vi "Convert Error Cluster to Table.vi"(11 "Error Codes":cluster{i32, string}[](array[cluster])) -> (2 "Code":i32[](array[numeric]), 3 "String":string[](array[string]))   [LabVIEW 2019, in "Diagnostics Addon System Explorer.lvlib"] (continued)
additional write network transactions can occur."}, {-40618, "LabVIEW: (Hex 0xFFFF6156) The reference is invalid."}, {-40616, "LabVIEW: (Hex 0xFFFF6158) The deterministic communication engine is unable to locate a device with a specified MAC address."}, {-40615, "LabVIEW: (Hex 0xFFFF6159) LabVIEW cannot instantiate the requested device in a specified mode because there is already a device initialized in deterministic mode."}, {-40613, "LabVIEW: (Hex 0xFFFF615B) The specified subchannel is out of range.  Refer to the LabVIEW Help for more information about supported ranges for channel subchannels."}, {-40612, "LabVIEW: (Hex 0xFFFF615C) You have attempted one of the following illegal operations: allocation of a write terminal on a channel that another node owns; allocation of a shared memory variable on a non-shared memory channel; creation of a read or write terminal on a shared memory channel."}, {-40611, "LabVIEW: (Hex 0xFFFF615D) An item with the specified index has already been configured."}, {-40609, "LabVIEW: (Hex 0xFFFF615F) The item offset is outside of the range you specified during channel initialization time."}, {-40608, "LabVIEW: (Hex 0xFFFF6160) One of the following occurred: 1) Message being written to the deterministic-communication engine exceeds the maximum size configured when the channel or terminal was created. 2) Buffer allocated for reading is smaller than the message size."}, {-40606, "LabVIEW: (Hex 0xFFFF6162) A timing source with the same name already exists for the deterministic-communication engine."}, {-40603, "LabVIEW: (Hex 0xFFFF6165) Files for the deterministic-communication engine are not installed properly."}, {-40602, "LabVIEW: (Hex 0xFFFF6166) Deterministic-communication engine ran out of allocated resources."}, {-40601, "LabVIEW: (Hex 0xFFFF6167) The deterministic-communication engine failed to initialize hardware."}, {-40600, "LabVIEW: (Hex 0xFFFF6168) The deterministic communication engine failed to allocate enough memory while performing the requested operation."}, {-36517, "LabVIEW: (Hex 0xFFFF715B) MathScript cannot execute a function which is overwritten by a variable in other code branches."}, {-36516, "LabVIEW: (Hex 0xFFFF715C) The variable is undefined. Assign a value to the variable before read access occurs."}, {-36515, "LabVIEW: (Hex 0xFFFF715D) Accessing a structure field is only supported for scalar structures but not for structure arrays."}, {-36514, "LabVIEW: (Hex 0xFFFF715E) Argument must be a positive integer scalar."}, {-36513, "LabVIEW: (Hex 0xFFFF715F) User-defined error message:"}, {-36512, "LabVIEW: (Hex 0xFFFF7160) Output data lost due to converting a non-vector character array to a string."}, {-36511, "LabVIEW: (Hex 0xFFFF7161) The result is not applicable because it returned a complex integer data type, which is not supported."}, {-36510, "LabVIEW: (Hex 0xFFFF7162) The switch selector must be a scalar."}, {-36509, "LabVIEW: (Hex 0xFFFF7163) The complete evaluation of a short-circuit expression detected a semantic error."}, {-36508, "LabVIEW: (Hex 0xFFFF7164) You must use an argument with a scalar value that can be converted into a logical value."}, {-36507, "LabVIEW: (Hex 0xFFFF7165) Converting a multi-element array into a scalar value resulted in lost output data."}, {-36506, "LabVIEW: (Hex 0xFFFF7166) Converting a complex number with non-zero imaginary values into a real number resulted in lost output data."}, {-36505, "LabVIEW: (Hex 0xFFFF7167) The argument types are not supported."}, {-36504, "LabVIEW: (Hex 0xFFFF7168) You cannot output an empty array as a scalar value."}, {-36503, "LabVIEW: (Hex 0xFFFF7169) The arguments must have matching dimensions to replace the indexing of an array."}, {-36502, "LabVIEW: (Hex 0xFFFF716A) The index is out of bounds."}, {-36501, "LabVIEW: (Hex 0xFFFF716B) The arguments must be positive integers or logicals."}, {-36500, "LabVIEW: (Hex 0xFFFF716C) The arguments must have matching dimensions to build an array."}, {-20339, "LabVIEW: (Hex 0xFFFFB08D) There must be a signal wired to each input signal terminal."}, {-10856, "LabVIEW: (Hex 0xFFFFD598) An unexpected error occurred from the operating system while performing the given operation."}, {-10846, "LabVIEW: (Hex 0xFFFFD5A2) Your application was unable to retrieve data from the background acquisition buffer fast enough so the unretrieved data was overwritten with new data.  To prevent this error, you might increase the size of the background acquisition buffer, increase the amount of data you read from it per call to the read function/VI, slow down your acquisition rate, or reduce the number of tasks your computer is performing."}, {-10804, "LabVIEW: (Hex 0xFFFFD5CC) The transfer stopped prior to reaching the end of the transfer buffer."}, {-10444, "LabVIEW: (Hex 0xFFFFD734) No more system memory is available on the heap, or no more memory is available on the device, or insufficient disk space is available."}, {-10408, "LabVIEW: (Hex 0xFFFFD758) The specified channel is in use."}, {-10405, "LabVIEW: (Hex 0xFFFFD75B) No channel is available."}, {-10403, "LabVIEW: (Hex 0xFFFFD75D) The specified device does not support the requested action (the driver recognizes the device, but the action is inappropriate for the device)."}, {-10402, "LabVIEW: (Hex 0xFFFFD75E) No device is located in the specified slot or at the specified address."}, {-10240, "LabVIEW: (Hex 0xFFFFD800) The driver interface could not locate or open the driver."}, {-10005, "LabVIEW: (Hex 0xFFFFD8EB) The device is invalid."}, {-10003, "LabVIEW: (Hex 0xFFFFD8ED) The value of a numeric parameter is invalid."}, {-4850, "LabVIEW: (Hex 0xFFFFED0E) Device driver not present or not supported."}, {-4824, "LabVIEW: (Hex 0xFFFFED28) Clipped Floating-point data to fit the range [-1.0, 1.0]."}, {-4820, "LabVIEW: (Hex 0xFFFFED2C) A buffer underflow has occurred."}, {-4803, "LabVIEW: (Hex 0xFFFFED3D) The sound driver or card does not support the specified operation."}, {-4702, "LabVIEW: (Hex 0xFFFFEDA2) One of the string parameters contains a null character. LabVIEW does not support null characters for regular expression matching."}, {-4701, "LabVIEW: (Hex 0xFFFFEDA3) The maximum recursion limit was reached while attempting the regular expression match"}, {-4644, "LabVIEW: (Hex 0xFFFFEDDC) An invalid UTF-8 string was used in a regular expression or input string."}, {-4643, "LabVIEW: (Hex 0xFFFFEDDD) Two named groups have the same name."}, {-4642, "LabVIEW: (Hex 0xFFFFEDDE) There is a syntax error after (?P."}, {-4641, "LabVIEW: (Hex 0xFFFFEDDF) An unrecognized character was encountered after (?P."}, {-4640, "LabVIEW: (Hex 0xFFFFEDE0) A recursive call could loop indefinitely."}, {-4639, "LabVIEW: (Hex 0xFFFFEDE1) Closing ) for (?C expected."}, {-4638, "LabVIEW: (Hex 0xFFFFEDE2) Number after (?C is > 255."}, {-4637, "LabVIEW: (Hex 0xFFFFEDE3) PCRE does not support \\L, \\l, \\N, \\P, \\p, \\U, \\u, or \\X escape sequences."}, {-4636, "LabVIEW: (Hex 0xFFFFEDE4) The \\C expression is not allowed in a lookbehind assertion."}, {-4635, "LabVIEW: (Hex 0xFFFFEDE5) Invalid condition (?(0)."}, {-4634, "LabVIEW: (Hex 0xFFFFEDE6) The character value in the \\x{...} sequence is too large."}, {-4632, "LabVIEW: (Hex 0xFFFFEDE8) UTF-8 is not supported."}, {-4631, "LabVIEW: (Hex 0xFFFFEDE9) POSIX collating elements are not supported."}, {-4630, "LabVIEW: (Hex 0xFFFFEDEA) Unknown POSIX class name."}, {-4629, "LabVIEW: (Hex 0xFFFFEDEB) A (?R or (?digits expression must be followed by )."}, {-4628, "LabVIEW: (Hex 0xFFFFEDEC) An assertion is expected after (?(."}, {-4627, "LabVIEW: (Hex 0xFFFFEDED) A conditional group contains more than two branches."}, {-4626, "LabVIEW: (Hex 0xFFFFEDEE) There is a malformed number after (?(."}, {-4625, "LabVIEW: (Hex 0xFFFFEDEF) A lookbehind assertion is not a fixed length."}, {-4624, "LabVIEW: (Hex 0xFFFFEDF0) The regular expression contains an unrecognized character after (?<."}, {-4623, "LabVIEW: (Hex 0xFFFFEDF1) Internal error: code overflow."}, {-4622, "LabVIEW: (Hex 0xFFFFEDF2) There is an unmatched parenthesis in a regular expression."}, {-4621, "LabVIEW: (Hex 0xFFFFEDF3) Failed to get the memory for regular expression matching."}, {-4620, "LabVIEW: (Hex 0xFFFFEDF4) The regular expression is too large."}, {-4619, "LabVIEW: (Hex 0xFFFFEDF5) Parentheses are nested too deeply."}, {-4618, "LabVIEW: (Hex 0xFFFFEDF6) A ) is missing after a comment."}, {-4617, "LabVIEW: (Hex 0xFFFFEDF7) Internal Error: Unknown option bit(s) set."}, {-4616, "LabVIEW: (Hex 0xFFFFEDF8) Internal Error: Erroffset passed as NULL."}, {-4615, "LabVIEW: (Hex 0xFFFFEDF9) There is a reference to non-existent subpattern."}, {-4614, "LabVIEW: (Hex 0xFFFFEDFA) A   ) is missing."}, {-4613, "LabVIEW: (Hex 0xFFFFEDFB) POSIX named classes are supported only within a class."}, {-4612, "LabVIEW: (Hex 0xFFFFEDFC) There is an unrecognized character after (?."}, {-4611, "LabVIEW: (Hex 0xFFFFEDFD) Internal error: unexpected repeat."}, {-4609, "LabVIEW: (Hex 0xFFFFEDFF) There is nothing to repeat."}, {-4608, "LabVIEW: (Hex 0xFFFFEE00) A range is out of order in a character class."}, {-4607, "LabVIEW: (Hex 0xFFFFEE01) A character class contains an invalid escape sequence."}, {-4606, "LabVIEW: (Hex 0xFFFFEE02) A character class is missing a ']' terminator."}, {-4605, "LabVIEW: (Hex 0xFFFFEE03) A number in the {} quantifier is too large."}, {-4604, "LabVIEW: (Hex 0xFFFFEE04) In the regular expression, the numbers within the quantifier {} are out of order."}, {-4603, "LabVIEW: (Hex 0xFFFFEE05) An unrecognized character follows a '\\'."}, {-4602, "LabVIEW: (Hex 0xFFFFEE06) A regular expression must not end with '\\c'. You must follow a '\\c' in a regular expression by another character to denote a control character."}, {-4601, "LabVIEW: (Hex 0xFFFFEE07) A regular expression must not end with '\\'."}, {-4600, "LabVIEW: (Hex 0xFFFFEE08) An unknown error occurred during the regular expression match."}, {-4550, "LabVIEW: (Hex 0xFFFFEE3A) This build specification uses VIs from a third party toolkit which is currently in evaluation mode."}, {-4502, "LabVIEW: (Hex 0xFFFFEE6A) A component of the given name is already loaded."}, {-4501, "LabVIEW: (Hex 0xFFFFEE6B) Cannot deploy without compiled code. Modify the build specification to include compiled code on the Additional Exclusions page before deploying."}, {-4407, "LabVIEW: (Hex 0xFFFFEEC9) LabVIEW cannot locate a palette item."}, {-4406, "LabVIEW: (Hex 0xFFFFEECA) A VI item in the <b>palette data</b> array is not supported in this version of LabVIEW."}, {-4404, "LabVIEW: (Hex 0xFFFFEECC) The value for <b>palette width</b> is invalid."}, {-4403, "LabVIEW: (Hex 0xFFFFEECD) A palette item is invalid."}, {-4402, "LabVIEW: (Hex 0xFFFFEECE) The palette view format is invalid."}, {-4401, "LabVIEW: (Hex 0xFFFFEECF) The specified file is not a valid palette file (.mnu)."}, {-4400, "LabVIEW: (Hex 0xFFFFEED0) The <b>palette type</b> is invalid."}, {-2985, "LabVIEW: (Hex 0xFFFFF457) The LabVIEW project is configured not to use source control. You must enable source control in order to perform source control operations."}, {-2984, "LabVIEW: (Hex 0xFFFFF458) The source control settings for the LabVIEW project require a different source control provider than what is configured for the LabVIEW environment. Select <b>Tools>>Source Control>>Configure Source Control</b> to change the source control provider for the LabVIEW environment."}, {-2983, "LabVIEW: (Hex 0xFFFFF459) LabVIEW could not access the source control provider. The LabVIEW source control configuration settings are not valid for this session or a timeout occurred. Select <b>Tools>>Source Control>>Configure Source Control</b> to reconfigure source control."}, {-2982, "LabVIEW: (Hex 0xFFFFF45A) The specified file is not a valid LabVIEW file type. Enter a path to an existing LabVIEW file, such as a VI or control."}, {-2981, "LabVIEW: (Hex 0xFFFFF45B) An error occurred while comparing the specified file. The local file is not the latest version in source control."}, {-2980, "LabVIEW: (Hex 0xFFFFF45C) The value of an input parameter is out of range."}, {-2979, "LabVIEW: (Hex 0xFFFFF45D) The source control configuration data is invalid, corrupted, or missing. Verify that the data is valid for the source control provider you selected during configuration."}, {-2978, "LabVIEW: (Hex 0xFFFFF45E) The number of files input does not match the version information input. Make sure the two inputs contain the same number of elements."}, {-2977, "LabVIEW: (Hex 0xFFFFF45F) The input file type is not compatible with the file retrieval method."}, {-2976, "LabVIEW: (Hex 0xFFFFF460) Invalid source control reference."}, {-2975, "LabVIEW: (Hex 0xFFFFF461) No valid file paths were specified. You must enter at least one valid file path."}, {-2974, "LabVIEW: (Hex 0xFFFFF462) An error occurred while uninitializing the source control provider."}, {-2973, "LabVIEW: (Hex 0xFFFFF463) An error occurred while loading the source control DLL. The source control provider might have been moved or removed without a registry update. You might need to reinstall the source control provider."}, {-2972, "LabVIEW: (Hex 0xFFFFF464) An internal error occurred during the source control operation."}, {-2971, "LabVIEW: (Hex 0xFFFFF465) An error occurred while accessing the source control provider. The specified provider was not found."}, {-2970, "LabVIEW: (Hex 0xFFFFF466) You cannot perform source control operations until you configure source control in LabVIEW. Select <b>Tools>>Source Control>>Configure Source Control</b> to configure source control."}, {-2964, "LabVIEW: (Hex 0xFFFFF46C) You cannot perform the specified source control operation on files marked as Open for Add or Open for Delete. Submit these files to the source control provider before you attempt the operation."}, {-2963, "LabVIEW: (Hex 0xFFFFF46D) The changelist does not include a valid description. Verify that the description is not empty and does not contain the default text."}, {-2962, "LabVIEW: (Hex 0xFFFFF46E) Unable to locate or run the administration tool from the source control provider."}, {-2961, "LabVIEW: (Hex 0xFFFFF46F) All files in a single submit operation must be the latest version, checked out to the user, not locked by another user, and under source control."}, {-2960, "LabVIEW: (Hex 0xFFFFF470) The specified files are not in the same changelist. All files in a single submit operation must be in the same changelist."}, {-2955, "LabVIEW: (Hex 0xFFFFF475) An error occurred during the specified source control operation."}, {-2954, "LabVIEW: (Hex 0xFFFFF476) A connection with the source control provider already exists. Disconnect from the current source control provider before you open a new connection."}, {-2953, "LabVIEW: (Hex 0xFFFFF477) The specified source control provider is not compatible with LabVIEW. The source control provider does not support required LabVIEW functionality."}, {-2952, "LabVIEW: (Hex 0xFFFFF478) The length of an input parameter exceeds the maximum allowed value."}, {-2951, "LabVIEW: (Hex 0xFFFFF479) The specified source control operation cannot run because the source control provider is not initialized."}, {-2950, "LabVIEW: (Hex 0xFFFFF47A) The specified option is invalid."}, {-2929, "LabVIEW: (Hex 0xFFFFF48F) A failure occurred in the connection with the source control provider."}, {-2928, "LabVIEW: (Hex 0xFFFFF490) Unable to locate the local copy of the specified file."}, {-2927, "LabVIEW: (Hex 0xFFFFF491) An error occurred while opening a source control project or accessing a file. An input value uses invalid file syntax."}, {-2926, "LabVIEW: (Hex 0xFFFFF492) The user is not allowed to perform this operation."}, {-2925, "LabVIEW: (Hex 0xFFFFF493) An error occurred while performing the specified operation. No source control project is open."}, {-2924, "LabVIEW: (Hex 0xFFFFF494) An error occurred while opening a source control project or accessing a file. The specified path is invalid."}, {-2923, "LabVIEW: (Hex 0xFFFFF495) An error occurred while opening the specified source control project. An input value uses invalid syntax for the source control project syntax."}, {-2922, "LabVIEW: (Hex 0xFFFFF496) The specified source control project is already open."}, {-2921, "LabVIEW: (Hex 0xFFFFF497) An error occurred while logging into the source code provider. The specified user login is invalid. Verify the login information you entered."}, {-2920, "LabVIEW: (Hex 0xFFFFF498) An error occurred within the source control provider program, such as shell failure."}, {-2919, "LabVIEW: (Hex 0xFFFFF499) An error occurred during file check-in. The specified file was automatically merged but was not checked in because you must resolve a merge conflict manually."}, {-2918, "LabVIEW: (Hex 0xFFFFF49A) An error occurred during file check-in. The specified file was automatically merged but was not checked in, pending user verification."}, {-2917, "LabVIEW: (Hex 0xFFFFF49B) An error occurred while adding a file to source control. The source control provider does not support the file type (binary or text)."}, {-2916, "LabVIEW: (Hex 0xFFFFF49C) The source control provider did not perform the specified operation."}, {-2915, "LabVIEW: (Hex 0xFFFFF49D) The source control provider returned a non-specific error. The specified operation was not performed."}, {-2914, "LabVIEW: (Hex 0xFFFFF49E) The source control provider does not support the specified operation."}, {-2913, "LabVIEW: (Hex 0xFFFFF49F) The version of the file you specified does not exist or was not specified correctly. Specify a valid version or date and time."}, {-2912, "LabVIEW: (Hex 0xFFFFF4A0) An error occurred while retrieving or removing the specified file. The file is currently checked out, so the provider is unable to retrieve or remove it."}, {-2911, "LabVIEW: (Hex 0xFFFFF4A1) The specified file is not under source control."}, {-2910, "LabVIEW: (Hex 0xFFFFF4A2) An error occurred while adding a file to source control. The specified file is in source control already."}, {-2909, "LabVIEW: (Hex 0xFFFFF4A3) File check-in did not occur because of a conflict error. Another user has checked in the file."}, {-2908, "LabVIEW: (Hex 0xFFFFF4A4) An error occurred while accessing source control. Check for network or contention problems."}, {-2907, "LabVIEW: (Hex 0xFFFFF4A5) An error occurred while checking out a file. The specified file is exclusively checked out by another user."}, {-2906, "LabVIEW: (Hex 0xFFFFF4A6) An error occurred while checking out a file. The specified file is locked."}, {-2905, "LabVIEW: (Hex 0xFFFFF4A7) An error occurred while checking out a file. The specified file already is checked out."}, {-2904, "LabVIEW: (Hex 0xFFFFF4A8) An error occurred while checking in or undoing the check out of a file. The specified file is not checked out to the current user."}, {-2903, "LabVIEW: (Hex 0xFFFFF4A9) An error occurred while opening the specified source control project. The source control provider could not create the source control project."}, {-2902, "LabVIEW: (Hex 0xFFFFF4AA) An error occurred while opening the specified source control project. The source control provider does not recognize the project name. Verify that the project name and location are correct."}, {-2901, "LabVIEW: (Hex 0xFFFFF4AB) An error occurred during source control provider initialization."}, {-2769, "LabVIEW: (Hex 0xFFFFF52F) The XPath expression must be a location path. Refer to the W3C XPath Web\nsite at http://www.w3.org/TR/xpath for more information about XPath\nsyntax and location paths."}, {-2768, "LabVIEW: (Hex 0xFFFFF530) The XPath expression does not conform to XPath syntax. Refer to the W3C\nXPath Web site at http://www.w3.org/TR/xpath for more information\nabout XPath syntax."}, {-2767, "LabVIEW: (Hex 0xFFFFF531) An error occurred while performing an XPath query. Refer to the W3C XPath\nWeb site at http://www.w3.org/TR/xpath for more information about\nXPath syntax."}, {-2766, "LabVIEW: (Hex 0xFFFFF532) Attempted to perform an XPath query with an invalid node refnum."}, {-2765, "LabVIEW: (Hex 0xFFFFF533) File already exists at the specified path."}, {-2764, "LabVIEW: (Hex 0xFFFFF534) Attempted to call Create Document with invalid document type."}, {-2763, "LabVIEW: (Hex 0xFFFFF535) Attempted to set the Loading External DTD flag on invalid document."}, {-2762, "LabVIEW: (Hex 0xFFFFF536) Attempted to get the Loading External DTD flag on invalid document."}, {-2761, "LabVIEW: (Hex 0xFFFFF537) Attempted to set Validate Schema Full Checking on invalid document."}, {-2760, "LabVIEW: (Hex 0xFFFFF538) Attempted to get Validate Schema Full Checking on invalid document."}, {-2759, "LabVIEW: (Hex 0xFFFFF539) Attempted to get System ID on invalid notation."}, {-2758, "LabVIEW: (Hex 0xFFFFF53A) Attempted to get Public ID on invalid notation."}, {-2757, "LabVIEW: (Hex 0xFFFFF53B) Attempted to call Replace Data on invalid character data."}, {-2756, "LabVIEW: (Hex 0xFFFFF53C) Attempted to call Delete Data on invalid character data."}, {-2755, "LabVIEW: (Hex 0xFFFFF53D) Attempted to call Insert Data on invalid character data."}, {-2754, "LabVIEW: (Hex 0xFFFFF53E) Attempted to call Append Data on invalid character data."}, {-2753, "LabVIEW: (Hex 0xFFFFF53F) Attempted to get Substring Data on invalid character data."}, {-2752, "LabVIEW: (Hex 0xFFFFF540) Attempted to get Length on invalid character data."}, {-2751, "LabVIEW: (Hex 0xFFFFF541) Attempted to set Data on invalid character data."}, {-2750, "LabVIEW: (Hex 0xFFFFF542) Attempted to get Data on invalid character data."}, {-2749, "LabVIEW: (Hex 0xFFFFF543) Attempted to call Has Attribute Namespace on invalid element."}, {-2748, "LabVIEW: (Hex 0xFFFFF544) Attempted to call Has Attribute on invalid element."}, {-2747, "LabVIEW: (Hex 0xFFFFF545) Attempted to call Get Element By Tag Name Namespace on invalid element."}, {-2746, "LabVIEW: (Hex 0xFFFFF546) Attempted to call Set Attribute Node Namespace with invalid parameter on element."}, {-2745, "LabVIEW: (Hex 0xFFFFF547) Attempted to call Set Attribute Node Namespace on invalid element."}, {-2744, "LabVIEW: (Hex 0xFFFFF548) Attempted to call Get Attribute Node Namespace on invalid element."}, {-2743, "LabVIEW: (Hex 0xFFFFF549) Attempted to call Remove Attribute Namespace on invalid element."}, {-2742, "LabVIEW: (Hex 0xFFFFF54A) Attempted to call Set Attribute Namespace on invalid element."}, {-2741, "LabVIEW: (Hex 0xFFFFF54B) Attempted to call Get Attribute Namespace on invalid element."}, {-2740, "LabVIEW: (Hex 0xFFFFF54C) Attempted to call Remove Attribute Node with invalid parameter on element."}, {-2739, "LabVIEW: (Hex 0xFFFFF54D) Attempted to call Remove Attribute Node on invalid element."}, {-2738, "LabVIEW: (Hex 0xFFFFF54E) Attempted to call Remove Attribute on invalid element."}, {-2737, "LabVIEW: (Hex 0xFFFFF54F) Attempted to call Set Attribute Node with invalid parameter on element."}, {-2736, "LabVIEW: (Hex 0xFFFFF550) Attempted to call Set Attribute Node on invalid element."}, {-2735, "LabVIEW: (Hex 0xFFFFF551) Attempted to call Set Attribute on invalid element."}, {-2734, "LabVIEW: (Hex 0xFFFFF552) Attempted to call Get Attribute Node on invalid element."}, {-2733, "LabVIEW: (Hex 0xFFFFF553) Attempted to get Attribute on invalid element."}, {-2732, "LabVIEW: (Hex 0xFFFFF554) Attempted to get Tag Name on invalid element."}, {-2731, "LabVIEW: (Hex 0xFFFFF555) Attempted to call Get Element By Tag Name on invalid element."}, {-2730, "LabVIEW: (Hex 0xFFFFF556) Attempted to get Item on invalid node list."}, {-2729, "LabVIEW: (Hex 0xFFFFF557) Attempted to get Length on invalid node list."}, {-2728, "LabVIEW: (Hex 0xFFFFF558) Attempted to get Length on invalid named node map."}, {-2727, "LabVIEW: (Hex 0xFFFFF559) Attempted to get Item on invalid named node map."}, {-2726, "LabVIEW: (Hex 0xFFFFF55A) Attempted to set Named Item Namespace with invalid parameter on named node map."}, {-2725, "LabVIEW: (Hex 0xFFFFF55B) Attempted to set Named Item Namespace on invalid named node map."}, {-2724, "LabVIEW: (Hex 0xFFFFF55C) Attempted to get Named Item Namespace on invalid named node map."}, {-2723, "LabVIEW: (Hex 0xFFFFF55D) Attempted to set Named Item with invalid parameter on named node map."}, {-2722, "LabVIEW: (Hex 0xFFFFF55E) Attempted to set Named Item on invalid named node map."}, {-2721, "LabVIEW: (Hex 0xFFFFF55F) Attempted to call Remove Named Item Namespace on invalid named node map."}, {-2720, "LabVIEW: (Hex 0xFFFFF560) Attempted to call Get Elements By ID on invalid document."}, {-2719, "LabVIEW: (Hex 0xFFFFF561) Attempted to call Get Elements By Tag Name Namespace on invalid document."}, {-2718, "LabVIEW: (Hex 0xFFFFF562) Attempted to call Create Attribute Namespace on invalid document."}, {-2717, "LabVIEW: (Hex 0xFFFFF563) Attempted to call Create Attribute Namespace with empty name string."}, {-2716, "LabVIEW: (Hex 0xFFFFF564) Attempted to call Create Element Namespace on invalid document."}, {-2715, "LabVIEW: (Hex 0xFFFFF565) Attempted to call Create Element Namespace with empty name string."}, {-2714, "LabVIEW: (Hex 0xFFFFF566) Attempted to set Do Schema on invalid document."}, {-2713, "LabVIEW: (Hex 0xFFFFF567) Attempted to get Do Schema on invalid document."}, {-2712, "LabVIEW: (Hex 0xFFFFF568) Error occurred while saving file because path is invalid."}, {-2711, "LabVIEW: (Hex 0xFFFFF569) Error occurred while loading file because path is invalid."}, {-2710, "LabVIEW: (Hex 0xFFFFF56A) Error occurred while loading file."}, {-2709, "LabVIEW: (Hex 0xFFFFF56B) Attempted to get Internal Subset on invalid DTD."}, {-2708, "LabVIEW: (Hex 0xFFFFF56C) Attempted to get System ID on invalid DTD."}, {-2707, "LabVIEW: (Hex 0xFFFFF56D) Attempted to get Public ID on invalid DTD."}, {-2706, "LabVIEW: (Hex 0xFFFFF56E) Attempted to call Create Document on invalid implementation."}, {-2705, "LabVIEW: (Hex 0xFFFFF56F) Attempted to call Create Document Type on invalid implementation."}, {-2704, "LabVIEW: (Hex 0xFFFFF570) Attempted to get Owner Element on invalid attribute."}, {-2703, "LabVIEW: (Hex 0xFFFFF571) Attempted to set Value on invalid attribute."}, {-2702, "LabVIEW: (Hex 0xFFFFF572) Attempted to get Value on invalid attribute."}, {-2701, "LabVIEW: (Hex 0xFFFFF573) Attempted to get Name on invalid attribute."}, {-2700, "LabVIEW: (Hex 0xFFFFF574) Attempted to call Is Supported on invalid node refnum."}, {-2699, "LabVIEW: (Hex 0xFFFFF575) Attempted to set Prefix on invalid node refnum."}, {-2698, "LabVIEW: (Hex 0xFFFFF576) Access to the XML parser must go through an initialized document."}, {-2697, "LabVIEW: (Hex 0xFFFFF577) Attempted to get Attributes with invalid parameter New Node."}, {-2696, "LabVIEW: (Hex 0xFFFFF578) Attempted to get Attributes on invalid named node map refnum."}, {-2695, "LabVIEW: (Hex 0xFFFFF579) Attempted to call Remove Named Item on invalid named node map."}, {-2694, "LabVIEW: (Hex 0xFFFFF57A) Attempted to get Named Item on invalid named node map."}, {-2693, "LabVIEW: (Hex 0xFFFFF57B) Attempted to get array on invalid named node map."}, {-2692, "LabVIEW: (Hex 0xFFFFF57C) Attempted to set Preserve Whitespace on invalid document."}, {-2691, "LabVIEW: (Hex 0xFFFFF57D) Attempted to get Preserve Whitespace on invalid document."}, {-2690, "LabVIEW: (Hex 0xFFFFF57E) Attempted to call Implementation on invalid document."}, {-2689, "LabVIEW: (Hex 0xFFFFF57F) Attempted to set Validate On Load on invalid document."}, {-2688, "LabVIEW: (Hex 0xFFFFF580) Attempted to get Validate On Load on invalid document."}, {-2687, "LabVIEW: (Hex 0xFFFFF581) Attempted to call Get Elements By Tag Name on invalid document."}, {-2686, "LabVIEW: (Hex 0xFFFFF582) Attempted to get DocType on invalid document."}, {-2685, "LabVIEW: (Hex 0xFFFFF583) Attempted to call Create Text Node on invalid document."}, {-2684, "LabVIEW: (Hex 0xFFFFF584) Attempted to call Create Document Fragment on invalid document."}, {-2683, "LabVIEW: (Hex 0xFFFFF585) Attempted to call Create Processing Instruction on invalid document."}, {-2682, "LabVIEW: (Hex 0xFFFFF586) Attempted to call Create Processing Instruction with empty target string."}, {-2681, "LabVIEW: (Hex 0xFFFFF587) Attempted to call Create Attribute on invalid document."}, {-2680, "LabVIEW: (Hex 0xFFFFF588) Attempted to call Create Attribute with empty name string."}, {-2679, "LabVIEW: (Hex 0xFFFFF589) Attempted to call Create CDATA Section on invalid document."}, {-2678, "LabVIEW: (Hex 0xFFFFF58A) Attempted to call Create Element on invalid document."}, {-2677, "LabVIEW: (Hex 0xFFFFF58B) Attempted to call Create Element with empty name string."}, {-2676, "LabVIEW: (Hex 0xFFFFF58C) Attempted to call Create Comment on invalid document."}, {-2675, "LabVIEW: (Hex 0xFFFFF58D) Attempted to get Document Element on invalid document."}, {-2674, "LabVIEW: (Hex 0xFFFFF58E) Attempted to call Save File on invalid document."}, {-2673, "LabVIEW: (Hex 0xFFFFF58F) Attempted to call Load File on invalid document."}, {-2672, "LabVIEW: (Hex 0xFFFFF590) Attempted to get Notations on invalid DTD."}, {-2671, "LabVIEW: (Hex 0xFFFFF591) Attempted to get Entities on invalid DTD."}, {-2670, "LabVIEW: (Hex 0xFFFFF592) Attempted to get Name on invalid DTD."}, {-2669, "LabVIEW: (Hex 0xFFFFF593) Attempted to call Has Feature on invalid implementation."}, {-2668, "LabVIEW: (Hex 0xFFFFF594) Attempted to get Notation Name on invalid entity."}, {-2667, "LabVIEW: (Hex 0xFFFFF595) Attempted to get System ID on invalid entity."}, {-2666, "LabVIEW: (Hex 0xFFFFF596) Attempted to get Public ID on invalid entity."}, {-2665, "LabVIEW: (Hex 0xFFFFF597) Attempted to set Data on invalid processing instruction."}, {-2664, "LabVIEW: (Hex 0xFFFFF598) Attempted to get Data on invalid processing instruction."}, {-2663, "LabVIEW: (Hex 0xFFFFF599) Attempted to get Target on invalid processing instruction."}, {-2662, "LabVIEW: (Hex 0xFFFFF59A) Attempted to call Split Text on invalid text node."}, {-2661, "LabVIEW: (Hex 0xFFFFF59B) Attempted to get Specified on invalid attribute."}, {-2660, "LabVIEW: (Hex 0xFFFFF59C) Attempted to call Replace Child with invalid node refnum parameter Old Child."}, {-2659, "LabVIEW: (Hex 0xFFFFF59D) Attempted to call Replace Child with invalid node refnum parameter New Child."}, {-2658, "LabVIEW: (Hex 0xFFFFF59E) Attempted to call Replace Child on invalid node refnum."}, {-2657, "LabVIEW: (Hex 0xFFFFF59F) Attempted to call Insert Before with invalid node refnum parameter New Child."}, {-2656, "LabVIEW: (Hex 0xFFFFF5A0) Attempted to call Insert Before on invalid node refnum."}, {-2655, "LabVIEW: (Hex 0xFFFFF5A1) Attempted to call Normalize on invalid node refnum."}, {-2654, "LabVIEW: (Hex 0xFFFFF5A2) Cannot call Normalize on node that is not of element type."}, {-2653, "LabVIEW: (Hex 0xFFFFF5A3) Attempted to call Get XML on invalid node refnum."}, {-2652, "LabVIEW: (Hex 0xFFFFF5A4) Attempted to call Has Child Nodes on invalid node refnum."}, {-2651, "LabVIEW: (Hex 0xFFFFF5A5) Attempted to call Clone Node on invalid node refnum."}, {-2648, "LabVIEW: (Hex 0xFFFFF5A8) Attempted to call Append Child with invalid refnum parameter New Child."}, {-2647, "LabVIEW: (Hex 0xFFFFF5A9) Attempted to call Append Child on invalid refnum."}, {-2646, "LabVIEW: (Hex 0xFFFFF5AA) Attempted to call Remove Child with invalid refnum parameter Old Child."}, {-2645, "LabVIEW: (Hex 0xFFFFF5AB) Attempted to call Remove Child on invalid node refnum."}, {-2644, "LabVIEW: (Hex 0xFFFFF5AC) Attempted to set Node Value on invalid node refnum."}, {-2643, "LabVIEW: (Hex 0xFFFFF5AD) Attempted to get Attributes on invalid node refnum."}, {-2642, "LabVIEW: (Hex 0xFFFFF5AE) Attempted to get Namespace Name on invalid node refnum."}, {-2641, "LabVIEW: (Hex 0xFFFFF5AF) Attempted to get Prefix Name on invalid node refnum."}, {-2640, "LabVIEW: (Hex 0xFFFFF5B0) Attempted to get Local Name on invalid node refnum."}, {-2639, "LabVIEW: (Hex 0xFFFFF5B1) Attempted to get Owner Document on invalid node refnum."}, {-2638, "LabVIEW: (Hex 0xFFFFF5B2) Attempted to get Previous Sibling on invalid node refnum."}, {-2637, "LabVIEW: (Hex 0xFFFFF5B3) Attempted to get Next Sibling on invalid node refnum."}, {-2636, "LabVIEW: (Hex 0xFFFFF5B4) Attempted to get Parent Node on invalid node refnum."}, {-2635, "LabVIEW: (Hex 0xFFFFF5B5) Attempted to get Last Child on invalid node refnum."}, {-2634, "LabVIEW: (Hex 0xFFFFF5B6) Attempted to get First Child on invalid node refnum."}, {-2633, "LabVIEW: (Hex 0xFFFFF5B7) Attempted to get Child Nodes on invalid node refnum."}, {-2632, "LabVIEW: (Hex 0xFFFFF5B8) Attempted to get Node Value on invalid node refnum."}, {-2631, "LabVIEW: (Hex 0xFFFFF5B9) Attempted to get Node Name on invalid node refnum."}, {-2630, "LabVIEW: (Hex 0xFFFFF5BA) Attempted to get Node Type on invalid node refnum."}, {-2629, "LabVIEW: (Hex 0xFFFFF5BB) An unknown error occurred."}, {-2628, "LabVIEW: (Hex 0xFFFFF5BC) An error occurred while parsing the document."}, {-2627, "LabVIEW: (Hex 0xFFFFF5BD) An unknown user error occurred."}, {-2626, "LabVIEW: (Hex 0xFFFFF5BE) Invalid refnum."}, {-2625, "LabVIEW: (Hex 0xFFFFF5BF) An error occurred while saving the document."}, {-2616, "LabVIEW: (Hex 0xFFFFF5C8) A system error occurred."}, {-2615, "LabVIEW: (Hex 0xFFFFF5C9) Operation not performed. Validation error. You used a method that would invalidate the node."}, {-2614, "LabVIEW: (Hex 0xFFFFF5CA) A parameter or operation was not supported by the underlying object."}, {-2613, "LabVIEW: (Hex 0xFFFFF5CB) Attempted to create or change an object in a way that was incorrect with regard to namespaces."}, {-2612, "LabVIEW: (Hex 0xFFFFF5CC) Attempted to modify the type of an underlying object."}, {-2611, "LabVIEW: (Hex 0xFFFFF5CD) Specified an invalid or illegal string."}, {-2610, "LabVIEW: (Hex 0xFFFFF5CE) Attempted to use an object that is no longer usable."}, {-2609, "LabVIEW: (Hex 0xFFFFF5CF) Attempted to add an attribute already in use."}, {-2608, "LabVIEW: (Hex 0xFFFFF5D0) Requested a type of object or operation that implementation does not support."}, {-2607, "LabVIEW: (Hex 0xFFFFF5D1) Attempted to reference a node in a context where it does not exist."}, {-2606, "LabVIEW: (Hex 0xFFFFF5D2) Attempted to modify an object where modifications are not allowed."}, {-2605, "LabVIEW: (Hex 0xFFFFF5D3) Specified data for a node that does not support data."}, {-2604, "LabVIEW: (Hex 0xFFFFF5D4) Specified an invalid or illegal character, possibly in a name."}, {-2603, "LabVIEW: (Hex 0xFFFFF5D5) Used a node in a document other than the one that created the node, and which does not support the node."}, {-2602, "LabVIEW: (Hex 0xFFFFF5D6) Inserted node in the wrong location."}, {-2601, "LabVIEW: (Hex 0xFFFFF5D7) Specified a range of text that does not fit into a string."}, {-2600, "LabVIEW: (Hex 0xFFFFF5D8) Index or size is negative or is greater than the allowed value."}, {-2595, "LabVIEW: (Hex 0xFFFFF5DD) Failed to get the version information about the DataPlugin."}, {-2594, "LabVIEW: (Hex 0xFFFFF5DE) An error occurred while connecting to the DataPlugin server. Possible reasons include a failed network connection or a server connection problem."}, {-2593, "LabVIEW: (Hex 0xFFFFF5DF) An error occurred while installing the DataPlugin. Possible reasons include an invalid DataPlugin name or a failed network connection."}, {-2592, "LabVIEW: (Hex 0xFFFFF5E0) TDMS does not support replacing channel values."}, {-2591, "LabVIEW: (Hex 0xFFFFF5E1) You must install NI-DAQmx on the computer to store NI-DAQmx properties by using the Storage/DataPlugin VIs."}, {-2590, "LabVIEW: (Hex 0xFFFFF5E2) Failed to export the DataPlugin. You can export only DataPlugins with a type of VBS or VBCrypt. Use the List DataPlugins VI to view the type of a DataPlugin."}, {-2589, "LabVIEW: (Hex 0xFFFFF5E3) Failed to unregister the DataPlugin. You cannot unregister the DataPlugins that LabVIEW installs by default."}, {-2588, "LabVIEW: (Hex 0xFFFFF5E4) Failed to register the DataPlugin. The DataPlugin .uri file might contain invalid DataPlugin information."}, {-2587, "LabVIEW: (Hex 0xFFFFF5E5) LabVIEW failed to write data to the .tdms file. Ensure that the <b>file format version</b> you specified for the TDMS Open function supports the data you want to write."}, {-2586, "LabVIEW: (Hex 0xFFFFF5E6) Support for the TDMS file format is not currently installed on your machine."}, {-2585, "LabVIEW: (Hex 0xFFFFF5E7) The .tdm file format is not currently supported on this operating system."}, {-2584, "LabVIEW: (Hex 0xFFFFF5E8) DIAdem could not be started. You must have DIAdem 9.1 Service Pack 2 or later installed to use the DIAdem Report Express VI."}, {-2583, "LabVIEW: (Hex 0xFFFFF5E9) Cannot append data to the existing file because the value of the X Value Columns option of the Write to Measurement File Express VI changed."}, {-2582, "LabVIEW: (Hex 0xFFFFF5EA) The Write to Measurement File Express VI cannot append new data to the file because the time information of the signals stored in the file does not match the signals you are trying to append."}, {-2581, "LabVIEW: (Hex 0xFFFFF5EB) The Write to Measurement File Express VI cannot append new data to the file because the signals stored in the file don't match the signals you are trying to append."}, {-2580, "LabVIEW: (Hex 0xFFFFF5EC) The Write to Measurement File Express VI cannot append new data to frequency domain waveforms."}, {-2578, "LabVIEW: (Hex 0xFFFFF5EE) After deleting data from a file, you must close the file and reopen it before you can perform a read operation."}, {-2575, "LabVIEW: (Hex 0xFFFFF5F1) Storage VIs version conflict."}, {-2574, "LabVIEW: (Hex 0xFFFFF5F2) The string you wired to this VI contains binary characters that are not valid entries for string values in a .tdm file. To store binary data, use data channels with a data type of 8-bit unsigned integer."}, {-2572, "LabVIEW: (Hex 0xFFFFF5F4) This property is not part of the Storage VI data structure."}, {-2571, "LabVIEW: (Hex 0xFFFFF5F5) This object type is not part of the Storage VI data structure."}, {-2570, "LabVIEW: (Hex 0xFFFFF5F6) LabVIEW could not write the file back to disk."}, {-2569, "LabVIEW: (Hex 0xFFFFF5F7) LabVIEW cannot convert the object ID into a valid refnum. An object with this ID does not exist in the data storage file."}, {-2568, "LabVIEW: (Hex 0xFFFFF5F8) LabVIEW failed to allocate memory from the operating system of your computer."}, {-2566, "LabVIEW: (Hex 0xFFFFF5FA) An input parameter to this VI is invalid."}, {-2565, "LabVIEW: (Hex 0xFFFFF5FB) LabVIEW could not load the data channel you specified from the data storage file. The channel either is empty or the properties that describe the channel, such as length or data type, are incomplete."}, {-2564, "LabVIEW: (Hex 0xFFFFF5FC) The software installed on this computer does not support the file format you requested. The Storage/DataPlugin VIs access files through plug-in libraries LabVIEW and DIAdem install."}, {-2563, "LabVIEW: (Hex 0xFFFFF5FD) This property does not exist."}, {-2562, "LabVIEW: (Hex 0xFFFFF5FE) The data type of a property or channel could not automatically be coerced when writing to or reading from a data storage file."}, {-2561, "LabVIEW: (Hex 0xFFFFF5FF) Data storage is write-protected."}, {-2560, "LabVIEW: (Hex 0xFFFFF600) LabVIEW cannot load the USI components the Storage/DataPlugin VIs require. These components are installed by LabVIEW and DIAdem."}, {-2559, "LabVIEW: (Hex 0xFFFFF601) The data storage file is already open."}, {-2558, "LabVIEW: (Hex 0xFFFFF602) LabVIEW cannot open the data storage file. Ensure that you chose a correct DataPlugin for this file format."}, {-2557, "LabVIEW: (Hex 0xFFFFF603) There is an error in the query expression."}, {-2556, "LabVIEW: (Hex 0xFFFFF604) LabVIEW cannot find the object type."}, {-2555, "LabVIEW: (Hex 0xFFFFF605) LabVIEW cannot write to a read-only data storage file."}, {-2554, "LabVIEW: (Hex 0xFFFFF606) LabVIEW does not support the data type of this property."}, {-2553, "LabVIEW: (Hex 0xFFFFF607) The object refnum is invalid. The node that returned this refnum might have encountered an error and did not return a valid refnum. The storage this refnum refers to might have closed before the call executed."}, {-2551, "LabVIEW: (Hex 0xFFFFF609) The property data type does not match."}, {-2550, "LabVIEW: (Hex 0xFFFFF60A) This property does not exist."}, {-2549, "LabVIEW: (Hex 0xFFFFF60B) Asynchronous reads from an earlier operation are still in progress. You cannot configure or start an asynchronous read unless the previous operation has been completed or stopped. You can stop asynchronous reads by using the TDMS Stop Asynchronous Reads function."}, {-2548, "LabVIEW: (Hex 0xFFFFF60C) Failed to write raw data to the .tdms file without channel information. Use the TDMS Set Channel Information function to specify the channel information for the raw data. The error may be caused by incorrect calling of TDMS Create Scaling Information VI. To call this VI with TDMS Advanced functions, only call the TDMS Set Channel Information function after any calls to the TDMS Create Scaling Information VI."}, {-2547, "LabVIEW: (Hex 0xFFFFF60D) LabVIEW failed to complete this operation. Verify that the values of both the <b>max asynchronous writes</b> input of the TDMS Configure Asynchronous Writes function and the <b>number of buffers</b> input of the TDMS Configure Asynchronous Reads function are less than 64. Also verify the array size of the <b>data</b> input of the TDMS Advanced Write function is below the maximum value. Refer to the LabVIEW Help for more information about using the TDMS Advanced Write function."}, {-2546, "LabVIEW: (Hex 0xFFFFF60E) Asynchronous reads or writes failed due to timeout. Increase the timeout value for the corresponding function."}, {-2545, "LabVIEW: (Hex 0xFFFFF60F) TDMS asynchronous mode is not initialized properly. Make sure the <b>enable asynchronous?</b> input of the TDMS Advanced Open function is TRUE. If you are writing data to a file, also make sure the TDMS Configure Asynchronous Writes function exists. If you are reading data from a file, also make sure that both the TDMS Configure Asynchronous Reads and the TDMS Start Asynchronous Reads functions exist."}, {-2544, "LabVIEW: (Hex 0xFFFFF610) With operating system buffering disabled, array sizes and file positions for the Advanced TDMS VIs and functions must be integer multiples of the hard disk sector size. Use the TDMS Advanced Open function to retrieve the sector size."}, {-2543, "LabVIEW: (Hex 0xFFFFF611) LabVIEW failed to open the .tdms file for raw data access. This error occurs if the file format version is 1.0 or if the file contains raw data that is not encoded in native-endian. Use the TDMS Defragment function and the TDMS Convert Format VI to convert the file to native-endian and version 2.0."}, {-2542, "LabVIEW: (Hex 0xFFFFF612) Files that contain DAQmx data samples cannot be processed by the TDMS Convert Format, TDMS Defragment, and TDMS Delete Data functions."}, {-2541, "LabVIEW: (Hex 0xFFFFF613) Failed to scale the data in the .tdms file. The NI TDMS component on your computer does not support the scale type. Upgrade the NI TDMS component to the latest version before reading the .tdms file."}, {-2540, "LabVIEW: (Hex 0xFFFFF614) Reading data that was streamed to a .tdms file by NI-DAQmx and data that was added to the file using a different application requires separate TDMS Read functions."}, {-2539, "LabVIEW: (Hex 0xFFFFF615) This file cannot be written to, because it is opened and locked by another thread or process. This typically happens when a file is written by a hardware driver, for example NI-DAQmx."}, {-2538, "LabVIEW: (Hex 0xFFFFF616) Failed to add scaling information to the TDMS object. This object contains scaling information that has already been applied."}, {-2537, "LabVIEW: (Hex 0xFFFFF617) Failed to convert the \"name\" property to TDMS file format version 2.0. In file format version 2.0, \"name\" must be a string."}, {-2536, "LabVIEW: (Hex 0xFFFFF618) LabVIEW failed to scale the data in the .tdms file. Ensure that this function supports the data type that you specify."}, {-2535, "LabVIEW: (Hex 0xFFFFF619) LabVIEW failed to create a scale for the .tdms file."}, {-2534, "LabVIEW: (Hex 0xFFFFF61A) The type of interleaved data is not supported by TDMS."}, {-2533, "LabVIEW: (Hex 0xFFFFF61B) LabVIEW failed to save the data in interleaved format because the data is either an analog waveform, a compressed digital table or waveform, or a 1D or 2D string array. LabVIEW saved the data in decimated format."}, {-2532, "LabVIEW: (Hex 0xFFFFF61C) Invalid group name and/or channel name."}, {-2531, "LabVIEW: (Hex 0xFFFFF61D) LabVIEW could not unload the TDMS file component."}, {-2530, "LabVIEW: (Hex 0xFFFFF61E) Failed to perform the operation on this .tdms file because pending data for this file exists. Use the TDMS Flush function to flush the data to disk."}, {-2529, "LabVIEW: (Hex 0xFFFFF61F) In TDMS files, channels in the same channel group must have unique names. You can provide unique channel names by using the \"channel name(s)\" input of the specified TDM Streaming Function. If you are using waveforms or the LabVIEW Express Dynamic Data Type, use the waveform attribute \"NI_UpdateChannelName\" to set a channel name."}, {-2526, "LabVIEW: (Hex 0xFFFFF622) LabVIEW dynamically calculates the value of this property. You cannot write any values to this property. This typically applies to properties like \"NI_ChannelLength\" or \"NI_DataType\"."}, {-2525, "LabVIEW: (Hex 0xFFFFF623) TDMS file data could not be converted into the specified data type."}, {-2524, "LabVIEW: (Hex 0xFFFFF624) You have attempted to open a TDM file.  Use the Read From Measurement File Express VI or the Storage/DataPlugin VIs to open this file."}, {-2522, "LabVIEW: (Hex 0xFFFFF626) This TDMS file is open as a read-only file.  Close the file before you open it for writing."}, {-2519, "LabVIEW: (Hex 0xFFFFF629) LabVIEW could not load the TDMS file component."}, {-2518, "LabVIEW: (Hex 0xFFFFF62A) The specified array dimension is not supported. The TDMS functions support only 1D or 2D arrays."}, {-2516, "LabVIEW: (Hex 0xFFFFF62C) LabVIEW could not create an index file for this TDMS file. The disk might be write protected. Without an index file, LabVIEW will not be able to open the TDMS file."}, {-2515, "LabVIEW: (Hex 0xFFFFF62D) When appending data to an existing data channel, the data types of the existing data and the new data did not match."}, {-2514, "LabVIEW: (Hex 0xFFFFF62E) This function does not accept the specified data type."}, {-2513, "LabVIEW: (Hex 0xFFFFF62F) LabVIEW does not support properties of the specified data type."}, {-2511, "LabVIEW: (Hex 0xFFFFF631) The specified TDMS file is corrupt."}, {-2510, "LabVIEW: (Hex 0xFFFFF632) This TDMS file complies with a new version of the TDMS format that is not supported by this version of LabVIEW."}, {-2509, "LabVIEW: (Hex 0xFFFFF633) LabVIEW no longer supports this version of the TDMS file format."}, {-2508, "LabVIEW: (Hex 0xFFFFF634) Invalid property."}, {-2507, "LabVIEW: (Hex 0xFFFFF635) Invalid group name and/or channel name."}, {-2506, "LabVIEW: (Hex 0xFFFFF636) LabVIEW failed to read data from the TDMS file."}, {-2505, "LabVIEW: (Hex 0xFFFFF637) LabVIEW failed to write data to the TDMS file."}, {-2504, "LabVIEW: (Hex 0xFFFFF638) LabVIEW failed to close the TDMS file."}, {-2503, "LabVIEW: (Hex 0xFFFFF639) Specified file does not comply with TDMS file format standards."}, {-2502, "LabVIEW: (Hex 0xFFFFF63A) String values are stored in TDMS files in utf8 unicode format. LabVIEW uses operating system functions to convert the unicode data, and one of these operating system functions has returned an error.  This error may indicate that you are using characters that are not supported within the language settings on your machine."}, {-2501, "LabVIEW: (Hex 0xFFFFF63B) Invalid TDMS file reference."}, {-2500, "LabVIEW: (Hex 0xFFFFF63C) Storage VIs internal error."}, {-2233, "LabVIEW: (Hex 0xFFFFF747) Unable to retrieve CPU load information. Verify that CPU load monitoring is enabled on the target."}, {-2232, "LabVIEW: (Hex 0xFFFFF748) The number of specified CPUs exceeds the number of CPUs available on the target."}, {-2231, "LabVIEW: (Hex 0xFFFFF749) The CPU pool settings are invalid. Each pool must contain at least 1 CPU."}, {-2230, "LabVIEW: (Hex 0xFFFFF74A) This VI is not supported on the current platform."}, {-2223, "LabVIEW: (Hex 0xFFFFF751) The Variable Client Support software required by the shared variable is missing or of the wrong version."}, {-2221, "LabVIEW: (Hex 0xFFFFF753) The variable RT FIFO write buffer is full."}, {-2220, "LabVIEW: (Hex 0xFFFFF754) The variable RT FIFO read buffer is empty."}, {-2211, "LabVIEW: (Hex 0xFFFFF75D) There was an attempt to create a Refnum to an existing RT FIFO using inconsistent Read/Write modes."}, {-2209, "LabVIEW: (Hex 0xFFFFF75F) The required RT FIFO DLL function is not bound."}, {-2208, "LabVIEW: (Hex 0xFFFFF760) This version of LabVIEW does not support waveforms in an RT FIFO."}, {-2207, "LabVIEW: (Hex 0xFFFFF761) Invalid waveform passed to the RT FIFO."}, {-2206, "LabVIEW: (Hex 0xFFFFF762) RT FIFO does not exist."}, {-2205, "LabVIEW: (Hex 0xFFFFF763) RT FIFO must contain at least two elements."}, {-2204, "LabVIEW: (Hex 0xFFFFF764) Type mismatch. The named RT FIFO type does not match the type of the existing RT FIFO with the same name."}, {-2203, "LabVIEW: (Hex 0xFFFFF765) Cannot match an empty name."}, {-2202, "LabVIEW: (Hex 0xFFFFF766) The specified name does not exist."}, {-2201, "LabVIEW: (Hex 0xFFFFF767) The specified name already exists and is of a different size or type."}, {-2200, "LabVIEW: (Hex 0xFFFFF768) Unknown internal error."}, {-1823, "LabVIEW: (Hex 0xFFFFF8E1) The input waveform has more signals than expected."}, {-1822, "LabVIEW: (Hex 0xFFFFF8E2) The input waveform has fewer signals than expected."}, {-1821, "LabVIEW: (Hex 0xFFFFF8E3) Waveform data type file datalog type conflict."}, {-1820, "LabVIEW: (Hex 0xFFFFF8E4) The t0 does not align with the end of the previous signal."}, {-1817, "LabVIEW: (Hex 0xFFFFF8E7) Specified start position or signal index is out of range."}, {-1816, "LabVIEW: (Hex 0xFFFFF8E8) Full Scale Range cannot be less than or equal to zero."}, {-1815, "LabVIEW: (Hex 0xFFFFF8E9) An invalid character was present in the spreadsheet string. Use only 0, 1, L, H, X, Z, V, or T."}, {-1813, "LabVIEW: (Hex 0xFFFFF8EB) Too many signals to convert into the specified data type."}, {-1812, "LabVIEW: (Hex 0xFFFFF8EC) Specified start position or duration is out of range."}, {-1811, "LabVIEW: (Hex 0xFFFFF8ED) Both waveforms must contain the same number of signals."}, {-1810, "LabVIEW: (Hex 0xFFFFF8EE) The number of samples to compare exceeds the number of samples after the start sample."}, {-1809, "LabVIEW: (Hex 0xFFFFF8EF) Highest resolution supported for conversion is 52."}, {-1808, "LabVIEW: (Hex 0xFFFFF8F0) Values other than 0, 1, L, H are present in the digital data."}, {-1807, "LabVIEW: (Hex 0xFFFFF8F1) Appending data with mismatched numbers of digital samples or signals."}, {-1806, "LabVIEW: (Hex 0xFFFFF8F2) Signal value input is outside the range of the digital data."}, {-1805, "LabVIEW: (Hex 0xFFFFF8F3) Start index out of range"}, {-1804, "LabVIEW: (Hex 0xFFFFF8F4) Start index, value, or tolerance is NaN"}, {-1803, "LabVIEW: (Hex 0xFFFFF8F5) Waveform x-axis value requested is out of range."}, {-1802, "LabVIEW: (Hex 0xFFFFF8F6) Waveforms have different dt values."}, {-1801, "LabVIEW: (Hex 0xFFFFF8F7) Duration input is not an integer multiple of dt. Value was coerced to nearest integer multiple of dt."}, {-1800, "LabVIEW: (Hex 0xFFFFF8F8) Start time input is not an integer multiple of dt. Value was coerced to nearest integer multiple of dt."}, {-1719, "LabVIEW: (Hex 0xFFFFF949) Index is out of range in a put operation."}, {-1718, "LabVIEW: (Hex 0xFFFFF94A) The contents of the reply you are accessing have not arrived yet."}, {-1717, "LabVIEW: (Hex 0xFFFFF94B) No handler in the dispatch tables fits the parameters to AEGetEventHandler or AEGetCoercionHandler."}, {-1716, "LabVIEW: (Hex 0xFFFFF94C) Unknown Apple Event address type."}, {-1715, "LabVIEW: (Hex 0xFFFFF94D) Handler did not get all required parameters."}, {-1714, "LabVIEW: (Hex 0xFFFFF94E) Wrong keyword for a special function."}, {-1713, "LabVIEW: (Hex 0xFFFFF94F) No user interaction allowed."}, {-1712, "LabVIEW: (Hex 0xFFFFF950) Apple Event timed out."}, {-1711, "LabVIEW: (Hex 0xFFFFF951) User cancelled out of wait loop for reply or receipt."}, {-1710, "LabVIEW: (Hex 0xFFFFF952) Invalid sending mode was passed."}, {-1709, "LabVIEW: (Hex 0xFFFFF953) AEResetTimer was passed an invalid reply parameter."}, {-1708, "LabVIEW: (Hex 0xFFFFF954) AEResetTimer was passed an invalid reply parameter."}, {-1707, "LabVIEW: (Hex 0xFFFFF955) The event is not an Apple Event."}, {-1706, "LabVIEW: (Hex 0xFFFFF956) Need a newer version of Apple Event Manager."}, {-1705, "LabVIEW: (Hex 0xFFFFF957) Operation involving a list item failed."}, {-1704, "LabVIEW: (Hex 0xFFFFF958) Not a valid descriptor record."}, {-1703, "LabVIEW: (Hex 0xFFFFF959) Wrong descriptor type."}, {-1702, "LabVIEW: (Hex 0xFFFFF95A) Data in an Apple Event could not be read."}, {-1701, "LabVIEW: (Hex 0xFFFFF95B) Descriptor record was not found."}, {-1700, "LabVIEW: (Hex 0xFFFFF95C) Data could not be coerced to the requested descriptor type."}, {-1622, "LabVIEW: (Hex 0xFFFFF9AA) Size of input points and initial conditions are not the same."}, {-1621, "LabVIEW: (Hex 0xFFFFF9AB) Size of input points and initial conditions are not the same."}, {-1620, "LabVIEW: (Hex 0xFFFFF9AC) Size of input points and initial conditions are not the same."}, {-1619, "LabVIEW: (Hex 0xFFFFF9AD) Size of input points and initial conditions are not the same."}, {-1618, "LabVIEW: (Hex 0xFFFFF9AE) Size of input points and initial conditions are not the same."}, {-1617, "LabVIEW: (Hex 0xFFFFF9AF) Size of input points and zeros-poles-gains are not the same."}, {-1616, "LabVIEW: (Hex 0xFFFFF9B0) Size of input points and transfer functions are not the same."}, {-1615, "LabVIEW: (Hex 0xFFFFF9B1) Size of input points and filter coefficients are not the same."}, {-1614, "LabVIEW: (Hex 0xFFFFF9B2) Size of input points, initial conditions and bounds are not the same."}, {-1613, "LabVIEW: (Hex 0xFFFFF9B3) Size of input points and initial conditions are not the same."}, {-1612, "LabVIEW: (Hex 0xFFFFF9B4) Size of input points and zeros-poles-gains are not the same."}, {-1611, "LabVIEW: (Hex 0xFFFFF9B5) Size of input points and transfer functions are not the same."}, {-1610, "LabVIEW: (Hex 0xFFFFF9B6) Size of input points and initial conditions are not the same."}, {-1609, "LabVIEW: (Hex 0xFFFFF9B7) Size of input points and initial conditions, and bounds are not the same."}, {-1608, "LabVIEW: (Hex 0xFFFFF9B8) Size of input points and initial conditions are not the same."}, {-1607, "LabVIEW: (Hex 0xFFFFF9B9) Upper limit<lower limit."}, {-1606, "LabVIEW: (Hex 0xFFFFF9BA) Switch off point is greater than switch on point."}, {-1605, "LabVIEW: (Hex 0xFFFFF9BB) Quantization interval negative."}, {-1604, "LabVIEW: (Hex 0xFFFFF9BC) Failure in discrete filter specification."}, {-1603, "LabVIEW: (Hex 0xFFFFF9BD) Ill-conditioned MIMO system."}, {-1602, "LabVIEW: (Hex 0xFFFFF9BE) Highest coefficient of a polynomial close to 0."}, {-1601, "LabVIEW: (Hex 0xFFFFF9BF) Numerator/denominator inconsistency."}, {-1600, "LabVIEW: (Hex 0xFFFFF9C0) Upper bound<lower bound."}, {-1524, "LabVIEW: (Hex 0xFFFFFA0C) The input vector of the user-defined membership function shape must be monotonic, increasing values in X and Y."}, {-1523, "LabVIEW: (Hex 0xFFFFFA0D) Incorrect number of rules."}, {-1522, "LabVIEW: (Hex 0xFFFFFA0E) Error loading fuzzy controller file."}, {-1521, "LabVIEW: (Hex 0xFFFFFA0F) Error opening fuzzy controller file."}, {-1519, "LabVIEW: (Hex 0xFFFFFA11) Consequence term not found."}, {-1518, "LabVIEW: (Hex 0xFFFFFA12) Incorrect number of fulfillment values."}, {-1517, "LabVIEW: (Hex 0xFFFFFA13) Incorrect number of active consequence terms."}, {-1516, "LabVIEW: (Hex 0xFFFFFA14) Antecedent variable name not found."}, {-1515, "LabVIEW: (Hex 0xFFFFFA15) Input is less than antecedance term x min."}, {-1514, "LabVIEW: (Hex 0xFFFFFA16) Input is greater than antecedance term x max."}, {-1512, "LabVIEW: (Hex 0xFFFFFA18) Number of inputs does not match number of antecedent variables."}, {-1511, "LabVIEW: (Hex 0xFFFFFA19) Antecedent variable used multiple times."}, {-1509, "LabVIEW: (Hex 0xFFFFFA1B) Incorrect number of consequent terms."}, {-1508, "LabVIEW: (Hex 0xFFFFFA1C) Incorrect number of consequent variables."}, {-1507, "LabVIEW: (Hex 0xFFFFFA1D) Incorrect number of antecedent terms."}, {-1506, "LabVIEW: (Hex 0xFFFFFA1E) Incorrect number of antecedent variables."}, {-1504, "LabVIEW: (Hex 0xFFFFFA20) Linguistic term x max cannot be less than x min."}, {-1503, "LabVIEW: (Hex 0xFFFFFA21) Linguistic term point(s) cannot be less than x min."}, {-1502, "LabVIEW: (Hex 0xFFFFFA22) Linguistic term point(s) are greater than x max."}, {-1501, "LabVIEW: (Hex 0xFFFFFA23) Linguistic term points are out of order."}, {-1300, "LabVIEW: (Hex 0xFFFFFAEC) Instrument-specific error."}, {-1236, "LabVIEW: (Hex 0xFFFFFB2C) Error interpreting instrument response."}, {-1223, "LabVIEW: (Hex 0xFFFFFB39) Instrument identification query failed."}, {-1210, "LabVIEW: (Hex 0xFFFFFB46) Parameter out of range."}, {-932, "LabVIEW: (Hex 0xFFFFFC5C) Destination port requires authentication."}, {-931, "LabVIEW: (Hex 0xFFFFFC5D) Location name is invalid."}, {-930, "LabVIEW: (Hex 0xFFFFFC5E) Service method is other than ppcServiceRealTime."}, {-928, "LabVIEW: (Hex 0xFFFFFC60) Invalid user reference number."}, {-927, "LabVIEW: (Hex 0xFFFFFC61) User's password is wrong."}, {-926, "LabVIEW: (Hex 0xFFFFFC62) PPCStart failed because destination did not have an inform pending."}, {-925, "LabVIEW: (Hex 0xFFFFFC63) An error has occurred in the network."}, {-924, "LabVIEW: (Hex 0xFFFFFC64) Unable to create a new userRefNum."}, {-923, "LabVIEW: (Hex 0xFFFFFC65) The default userRefNum does not yet exist."}, {-922, "LabVIEW: (Hex 0xFFFFFC66) User has not specified owner name in Sharing Setup Control Panel."}, {-919, "LabVIEW: (Hex 0xFFFFFC69) PPCPortRec is invalid."}, {-917, "LabVIEW: (Hex 0xFFFFFC6B) The session has closed."}, {-916, "LabVIEW: (Hex 0xFFFFFC6C) The port was closed."}, {-915, "LabVIEW: (Hex 0xFFFFFC6D) Unable to contact destination application."}, {-914, "LabVIEW: (Hex 0xFFFFFC6E) A system resource is missing."}, {-913, "LabVIEW: (Hex 0xFFFFFC6F) User has not named his Macintosh in the Network Setup Control Panel."}, {-912, "LabVIEW: (Hex 0xFFFFFC70) Destination rejected the session request."}, {-911, "LabVIEW: (Hex 0xFFFFFC71) User name unknown on destination machine."}, {-910, "LabVIEW: (Hex 0xFFFFFC72) Another port is already open with this name (perhaps in another application)."}, {-909, "LabVIEW: (Hex 0xFFFFFC73) Bad parameter or invalid state for this operation."}, {-908, "LabVIEW: (Hex 0xFFFFFC74) Invalid session reference number."}, {-907, "LabVIEW: (Hex 0xFFFFFC75) PPC Toolbox is unable to create a session."}, {-906, "LabVIEW: (Hex 0xFFFFFC76) Port does not exist at destination."}, {-905, "LabVIEW: (Hex 0xFFFFFC77) Network activity is currently disabled."}, {-904, "LabVIEW: (Hex 0xFFFFFC78) The system is unable to allocate memory. This is a critical error, and you should restart."}, {-903, "LabVIEW: (Hex 0xFFFFFC79) Invalid port name. Unable to open port or bad portRefNum."}, {-902, "LabVIEW: (Hex 0xFFFFFC7A) Invalid or inappropriate locationKindSelector in locationName."}, {-900, "LabVIEW: (Hex 0xFFFFFC7C) PPC Toolbox has not been initialized."}, {-843, "LabVIEW: (Hex 0xFFFFFCB5) Cannot load Nanosecond Engine Dynamic Library."}, {-842, "LabVIEW: 
